vi "Get_Folder_Details.vi"(0 "Path":path, 11 "Error_In":errorcluster) -> (3 "Directory":bool, 4 "Path_Out":path, 6 "Parent_Path":path, 8 "Filename":string, 10 "Size":string, 15 "Error_Out":errorcluster)   [LabVIEW 2023, in "File_Handler_Library.lvlib"]
doc: "This VI get folder details"
uses:
  File_Handler_Library.lvlib
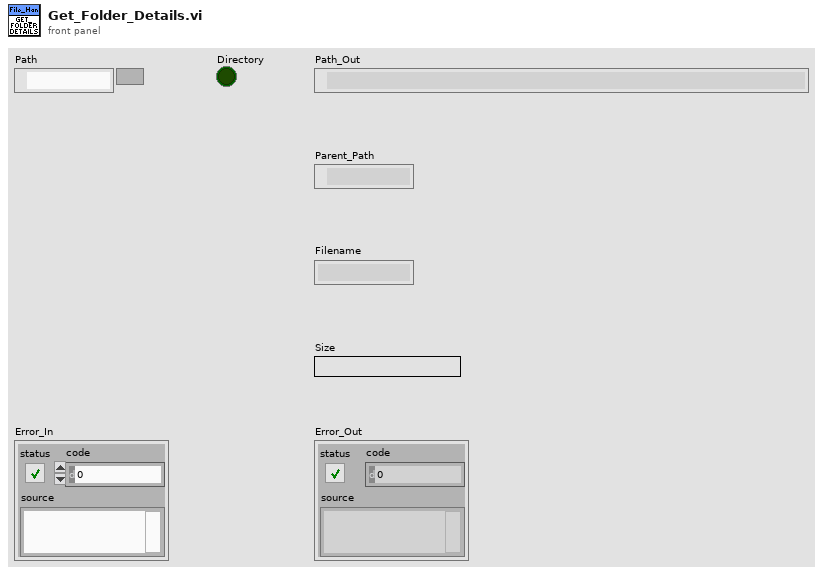
[diagram p1: front panel]
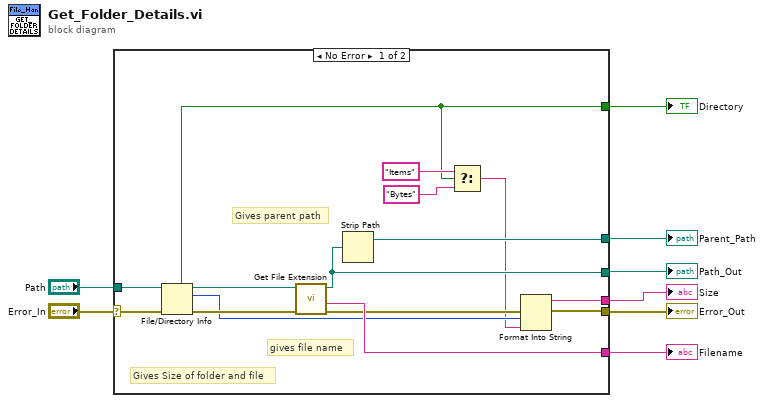
[diagram p0: block diagram]
diagram:
  n1 = case shown="No Error" "Error_In" {
    selector: "Error_In" -> [w23 w25]
    tunnel: "Path" -> [w22 w24]
    tunnel: [w14 _] -> w2
    tunnel: [w21 _] -> w6
    tunnel: [w18 w24] -> w5
    tunnel: [w11 w25] -> w4
    tunnel: [w17 _] -> w3
    tunnel: [w9 _] -> w1
    frame No Error {
      # "Gives parent path"
      # "gives file name"
      # "Gives Size of folder and file"
      n2 = File/Directory Info(path=w22, error in=w23) -> (path out=w19:path, directory=w14:bool, size=w13:i64, error out=w20:errorcluster)  [unwired: 3 out]
      n3 = call <vilib>:"Get File Extension.vi"("error in (no error)"=w20, "file"=w19) -> ("error out"=w12:errorcluster, "filename without extension"=w21:string, "dup file"=w18:path)  [unwired: 5 in, 2 out]
      n4 = Strip Path(path=w18) -> (stripped path=w17:path)  [unwired: 1 out]
      n5 = Select(t="Items", s=w14, f="Bytes") -> (s? t:f=w10:string)
      n6 = Format Into String(error in=w12, w13, w10) -> (resulting string=w9:string, error out=w11:errorcluster)  [unwired: 2 in]
    }
    frame Error {
    }
  }
  "Size" <- w1
  "Error_Out" <- w4
  "Path_Out" <- w5
  "Directory" <- w2
  "Filename" <- w6
  "Parent_Path" <- w3
